vi "NI-DCPower Pulse Current Sequence T9.vi"() -> ()   [LabVIEW 2021, in "DC POwer T9.lvlib"]
doc: "Demonstrates how to use the DCPower Pulse API to generate a Current Pulse Sequence. This example initializes a session, configures the Source Mode and the Output Function, configures the pulse parameters, initiates the pulse output sequence, and takes measurements. Refer to the Pulsing page in NI-DC Power Supplies and SMUs Help for additional information."
uses:
  DC POwer T9.lvlib
  <instrlib>/niDCPower/nidcpower.llb/niDCPower Source Mode.ctl
  <instrlib>/niDCPower/nidcpower.llb/niDCPower Aperture Time Units.ctl
  <instrlib>/niDCPower/nidcpower.llb/niDCPower Output Function.ctl
  <instrlib>/niDCPower/nidcpower.llb/niDCPower Wait For Event - Event.ctl
panel:
  in  "Pulse Current Level Range":dbl=1.0 format="%#.3p"
  in  "Pulse Bias Current Level":dbl format="%.5p"
  in  "Pulse Voltage Limit":dbl=1.0 format="%.5p"
  in  "Pulse Voltage Limit Range":dbl=1.0 format="%#.3p"
  in  "Pulse Bias Voltage Limit":dbl=1.0 format="%.5p"
  in  "Pulse Current Sequence":dbl[](array[numeric])=[0.1, 0.2, 0.3, 0.4]
  in  "Source Delays":dbl[](array[numeric])=[5e-05, 6e-05, 7e-05, 8e-05] format="%.3p"
  in  "Aperture Time (Sec)":dbl=0.0001
  out "Current Measurements":dbl[](array[numeric])
  out "Voltage Measurements":dbl[](array[numeric])
  in  "Pulse Bias Delay (Sec)":dbl=1e-06 format="%.5p"
  in  "Pulse Off Time (Sec)":dbl=0.005
  in  "Pulse On Time (Sec)":dbl=0.001
  in  "Source SMU":refnum<k15>="Dev1"
  in  "Source SMU Channel":string="0"
  # "Overview: This example outputs a sequence of current pulses and takes a voltage and current measurement at the peak of each pulse. \nRequirements: NI-DCPower\nInstructions:\n1. Select the appropriate device in the Resource Name control.\n2. Configure the pulse sequence that you would like to output.\n3. Run the VI."
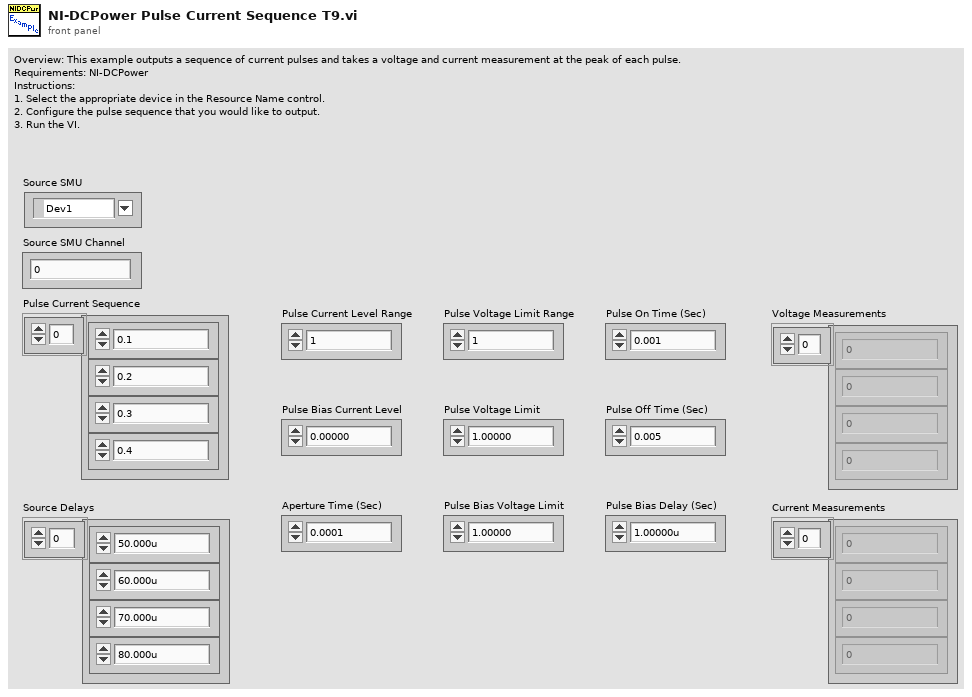
[diagram p1: front panel]
types:
  T1 = typedef "niDCPower Wait For Event - Event.ctl" = i32
  T2 = typedef "niDCPower Output Function.ctl" = i32
  T3 = typedef "niDCPower Aperture Time Units.ctl" = i32
  T4 = typedef "niDCPower Source Mode.ctl" = i32
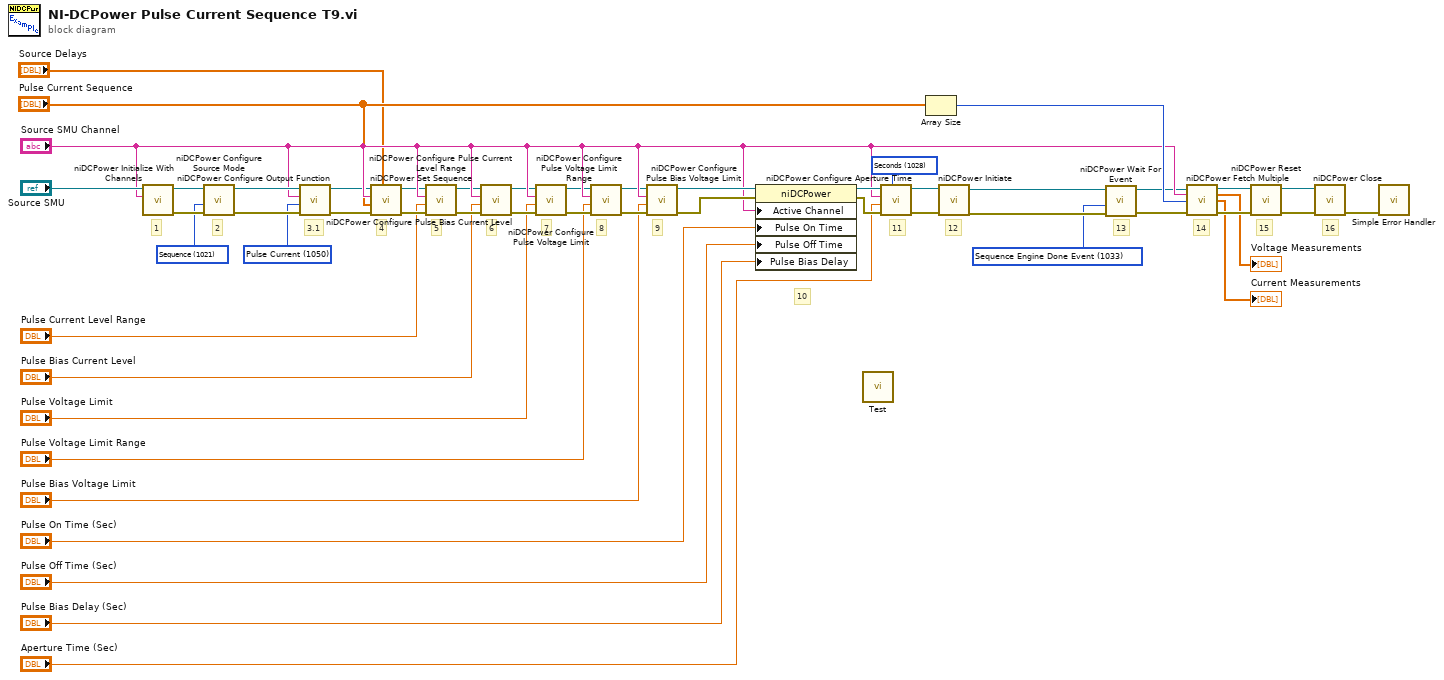
[diagram p0: block diagram]
diagram:
  w1 = T1 1033 items=["Source Complete Event"=1030, "Measure Complete Event"=1031, "Sequence Iteration Complete Event"=1032, "Sequence Engine Done Event"=1033, "Pulse Complete Event"=1051, "Ready For Pulse Trigger Event"=1052] ("event")
  w15 = T2 1050 items=["DC Voltage"=1006, "DC Current"=1007, "Pulse Voltage"=1049, "Pulse Current"=1050] ("output function")
  w28 = T3 1028 items=["Seconds"=1028, "Powerline Cycles"=1029] ("aperture time units")
  w47 = T4 1021 items=["Single Point"=1020, "Sequence"=1021] ("source mode")
  # "16"
  # "9"
  # "8"
  # "7"
  # "6"
  # "5"
  # "4"
  # "3.1"
  # "15"
  # "14"
  # "13"
  # "12"
  # "11"
  # "10"
  # "2"
  # "1"
  n1 = call <instrlib>:"niDCPower Initialize With Channels.vi"("channels"="Source SMU Channel", "resource name"="Source SMU") -> ("error out"=w51:errorcluster, "instrument handle out"=w44:refnum<k15>)  [unwired: 3 in, 5 out]
  n2 = call <instrlib>:"niDCPower Configure Source Mode.vi"("error in (no error)"=w51, "source mode"=w47, "instrument handle"=w44) -> ("error out"=w45:errorcluster, "instrument handle out"=w46:refnum<k15>)  [unwired: 7 out]
  n3 = call <instrlib>:"niDCPower Configure Output Function.vi"("error in (no error)"=w45, "output function"=w15, "channel name"="Source SMU Channel", "instrument handle"=w46) -> ("error out"=w9:errorcluster, "instrument handle out"=w8:refnum<k15>)  [unwired: 6 out]
  n4 = call <instrlib>:"niDCPower Set Sequence.vi"("source delays"="Source Delays", "error in (no error)"=w9, "values"="Pulse Current Sequence", "channel name"="Source SMU Channel", "instrument handle"=w8) -> ("error out"=w24:errorcluster, "instrument handle out"=w7:refnum<k15>)  [unwired: 5 in]
  n5 = call <instrlib>:"niDCPower Configure Pulse Current Level Range.vi"("error in (no error)"=w24, "pulse current level range"="Pulse Current Level Range", "channel name"="Source SMU Channel", "instrument handle"=w7) -> ("error out"=w23:errorcluster, "instrument handle out"=w22:refnum<k15>)  [unwired: 6 in]
  n6 = call <instrlib>:"niDCPower Configure Pulse Bias Current Level.vi"("error in (no error)"=w23, "pulse bias current level"="Pulse Bias Current Level", "channel name"="Source SMU Channel", "instrument handle"=w22) -> ("error out"=w21:errorcluster, "instrument handle out"=w20:refnum<k15>)  [unwired: 6 in]
  n7 = call <instrlib>:"niDCPower Configure Pulse Voltage Limit.vi"("error in (no error)"=w21, "pulse voltage limit"="Pulse Voltage Limit", "channel name"="Source SMU Channel", "instrument handle"=w20) -> ("error out"=w19:errorcluster, "instrument handle out"=w18:refnum<k15>)  [unwired: 6 in]
  n8 = call <instrlib>:"niDCPower Configure Pulse Voltage Limit Range.vi"("error in (no error)"=w19, "pulse voltage limit range"="Pulse Voltage Limit Range", "channel name"="Source SMU Channel", "instrument handle"=w18) -> ("error out"=w17:errorcluster, "instrument handle out"=w16:refnum<k15>)  [unwired: 6 in]
  n9 = call <instrlib>:"niDCPower Configure Pulse Bias Voltage Limit.vi"("error in (no error)"=w17, "pulse bias voltage limit"="Pulse Bias Voltage Limit", "channel name"="Source SMU Channel", "instrument handle"=w16) -> ("error out"=w38:errorcluster, "instrument handle out"=w39:refnum<k15>)  [unwired: 6 in]
  n10 = property class="niDCPower"(reference=w39, error in=w38, "Active Channel"="Source SMU Channel", "Pulse On Time"="Pulse On Time (Sec)", "Pulse Off Time"="Pulse Off Time (Sec)", "Pulse Bias Delay"="Pulse Bias Delay (Sec)") -> (reference out=w30:refnum<k15>, error out=w32:errorcluster)
  n11 = call "Test.vi"() -> ()  [unwired: 16 in]
  n12 = call <instrlib>:"niDCPower Configure Aperture Time.vi"("aperture time units"=w28, "error in (no error)"=w32, "aperture time"="Aperture Time (Sec)", "channel name"="Source SMU Channel", "instrument handle"=w30) -> ("error out"=w31:errorcluster, "instrument handle out"=w29:refnum<k15>)  [unwired: 5 in]
  n13 = Array Size(array="Pulse Current Sequence") -> (size(s)=w33:i32)
  n14 = call <instrlib>:"niDCPower Initiate.vi"("error in (no error)"=w31, "instrument handle"=w29) -> ("error out"=w4:errorcluster, "instrument handle out"=w5:refnum<k15>)  [unwired: 2 in, 6 out]
  n15 = call <instrlib>:"niDCPower Wait For Event.vi"("error in (no error)"=w4, "event"=w1, "instrument handle"=w5) -> ("error out"=w2:errorcluster, "instrument handle out"=w3:refnum<k15>)  [unwired: 7 in]
  n16 = call <instrlib>:"niDCPower Fetch Multiple.vi"("instrument handle"=w3, "channel name"="Source SMU Channel", "count (1)"=w33, "error in (no error)"=w2) -> ("instrument handle out"=w35:refnum<k15>, "voltage measurements"=→"Voltage Measurements":dbl[], "current measurements"=→"Current Measurements":dbl[], "error out"=w50:errorcluster)  [unwired: 6 in, 2 out]
  n17 = call <instrlib>:"niDCPower Reset.vi"("error in (no error)"=w50, "instrument handle"=w35) -> ("error out"=w42:errorcluster, "instrument handle out"=w41:refnum<k15>)  [unwired: 2 in, 6 out]
  n18 = call <instrlib>:"niDCPower Close.vi"("error in (no error)"=w42, "instrument handle"=w41) -> ("error out"=w43:errorcluster)  [unwired: 9 out]
  n19 = call <vilib>:"Simple Error Handler.vi"("error in (no error)"=w43) -> ()  [unwired: 1 in, 8 out]
